vi "SourceAllInfo.vi"(3 "COM Port in":refnum<visa-resource-name>, 9 "error in (no error)":errorcluster) -> (0 "COM Port out":refnum<visa-resource-name>, 6 "error out":errorcluster, 7 "Intensity":i32[](array[numeric]))   [LabVIEW 2009]
panel:
  out "Type":i32[](array[numeric])
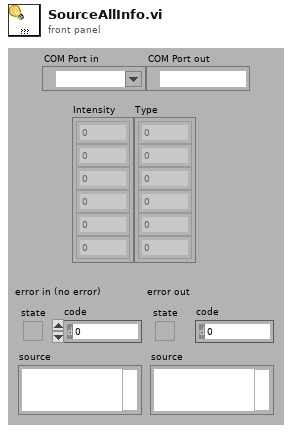
[diagram p1: front panel]
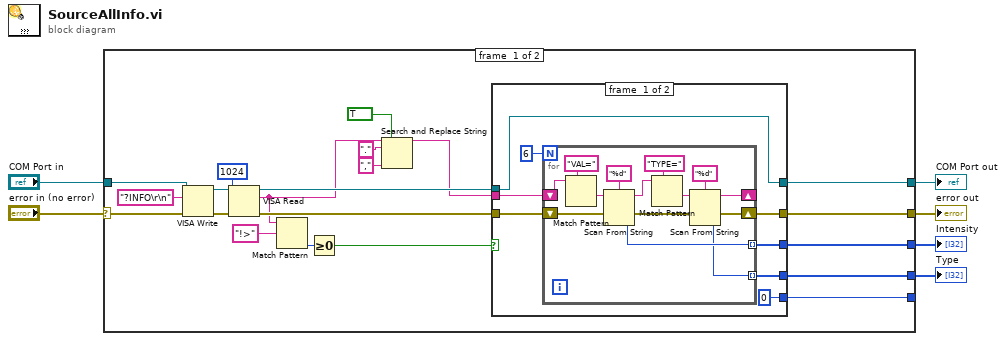
[diagram p0: block diagram]
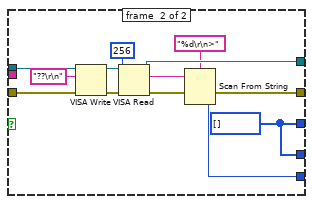
[diagram p2: hidden frame]
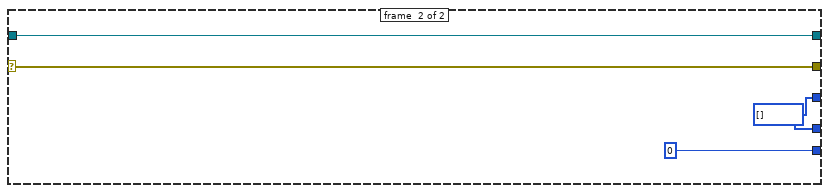
[diagram p3: hidden frame]
diagram:
  n1 = case shown="No Error" "error in (no error)" {
    selector: "error in (no error)" -> [w25 w66]
    tunnel: "COM Port in" -> [w27 w65]
    tunnel: [w18 w65] -> w3
    tunnel: [w17 w66] -> w4
    tunnel: [w14 0] -> _
    tunnel: [w13 w63] -> w2
    tunnel: [w7 w63] -> w1
    frame #0 {
      n2 = VISA Write(VISA resource name=w27, write buffer="?INFO\r\n", error in (no error)=w25) -> (VISA resource name out=w21:refnum<visa-resource-name>, error out=w22:errorcluster)  [unwired: 1 out]
      n3 = VISA Read(VISA resource name=w21, byte count=u32 1024 ("nombre d'octets (0)"), error in (no error)=w22) -> (VISA resource name out=w20:refnum<visa-resource-name>, read buffer=w12:string, error out=w19:errorcluster)  [unwired: 1 out]
      n4 = Match Pattern(string=w12, regular expression="!>") -> (offset past match=w23:i32)  [unwired: 4 out]
      n5 = Greater Or Equal To 0?(x=w23) -> (x >= 0?=w15:bool)
      n6 = Search and Replace String(replace all?=TRUE ("tout remplacer ? (F)"), input string=w12, search string="." ("chaîne recherchée"), replace string="," ("chaîne de remplacement (\"\")")) -> (result string=w11:string)  [unwired: 1 in, 6 out]
      n7 = case "Structure Condition" shown="False" w15 {
        tunnel: w19 -> [w32 w62]
        tunnel: w20 -> [w30 w61]
        tunnel: [w31 w52] -> w17
        tunnel: [w30 w56] -> w18
        tunnel: [0 w51] -> w14
        tunnel: w11 -> [w34 _]
        tunnel: [w29 w50] -> w13
        tunnel: [w28 w50] -> w7
        frame #0 {
          n8 = for {
            N: 6 -> [_]
            shift-right: [w36] -> _
            shift-left: w34 -> [w49]
            shift-right: [w38] -> w31
            shift-left: w32 -> [w47]
            tunnel: [w44] -> w29 mode=indexing
            tunnel: [w37] -> w28 mode=indexing
            n9 = Match Pattern(string=w49, regular expression="VAL=" ("expression régulière")) -> (after substring=w46:string)  [unwired: 4 out]
            n10 = Scan From String(format string="%d" ("chaîne de format"), input string=w46, error in=w47) -> (remaining string=w40:string, error out=w39:errorcluster, output 1=w44:i32)  [unwired: 1 in, 2 out]
            n11 = Match Pattern(string=w40, regular expression="TYPE=" ("expression régulière")) -> (after substring=w43:string)  [unwired: 4 out]
            n12 = Scan From String(format string="%d" ("chaîne de format"), input string=w43, error in=w39) -> (remaining string=w36:string, error out=w38:errorcluster, output 1=w37:i32)  [unwired: 1 in, 2 out]
          }
        }
        frame #1 {
          w50 = i32[] []
          n13 = VISA Write(VISA resource name=w61, write buffer="??\r\n" ("buffer à écrire"), error in (no error)=w62) -> (VISA resource name out=w57:refnum<visa-resource-name>, error out=w58:errorcluster)  [unwired: 1 out]
          n14 = VISA Read(VISA resource name=w57, byte count=u32 256 ("nombre d'octets (0)"), error in (no error)=w58) -> (VISA resource name out=w56:refnum<visa-resource-name>, read buffer=w53:string, error out=w54:errorcluster)  [unwired: 1 out]
          n15 = Scan From String(format string="%d\r\n>" ("chaîne de format"), input string=w53, error in=w54) -> (error out=w52:errorcluster, output 1=w51:i32)  [unwired: 1 in, 3 out]
        }
      }
    }
    frame #1 {
      w63 = i32[] []
    }
  }
  "Intensity" <- w2
  "error out" <- w4
  "COM Port out" <- w3
  "Type" <- w1
